vi "Cycling_No_DAQ_Tasks_No_cRio.vi"() -> ()   [LabVIEW 2020]
uses:
  Drivers-IT-M3400/IT-M3400.lvlib
panel:
  in  "Output Safety":T1
  in  "Number of Cycles":i32
  in  "Charge filepath":path
  in  "Discharge filepath":path
  in  "Batteryname":string
  in  "Starting Cycle":i32
  out "PS error out":errorcluster
  out "PS Visa Out":refnum<visa-resource-name>
  in  "Wait time":dbl
  in  "Discharge Current Setpoint":dbl format="%#.6g"
  in  "Charge Current Setpoint":dbl format="%#.6g"
  in  "Battery Type":T2(ring)
  in  "PS type":enum16{"NHR", "ITECH"}(ring)
  in  "PS error in":errorcluster caption="PS error in (no error)"
  in  "PS VISA in":refnum<visa-resource-name>
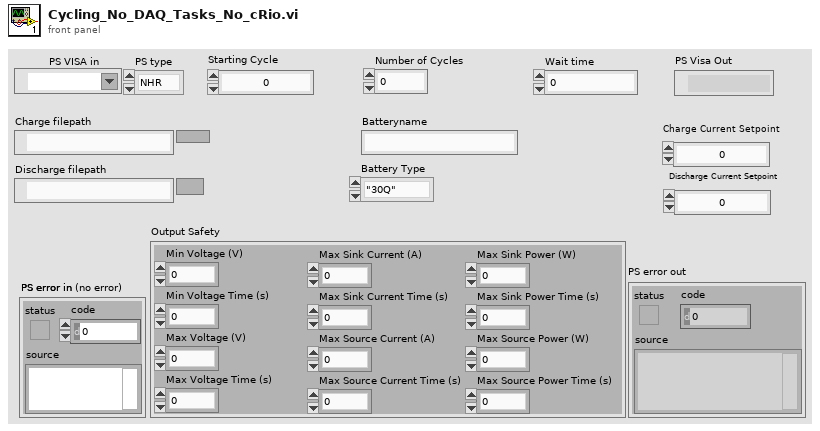
[diagram p1: front panel]
types:
  T1 = cluster{"Min Voltage (V)":dbl, "Min Voltage Time (s)":dbl, "Max Voltage (V)":dbl, "Max Voltage Time (s)":dbl, "Max Sink Current (A)":dbl, "Max Sink Current Time (s)":dbl, "Max Source Current (A)":dbl, "Max Source Current Time (s)":dbl, "Max Sink Power (W)":dbl, "Max Sink Power Time (s)":dbl, "Max Source Power (W)":dbl, "Max Source Power Time (s)":dbl}
  T2 = enum16{"\"30Q\"", "\"40T\"", "\"2P30Q\"", "\"3P30Q\"", "\"Nissan Leaf\""}
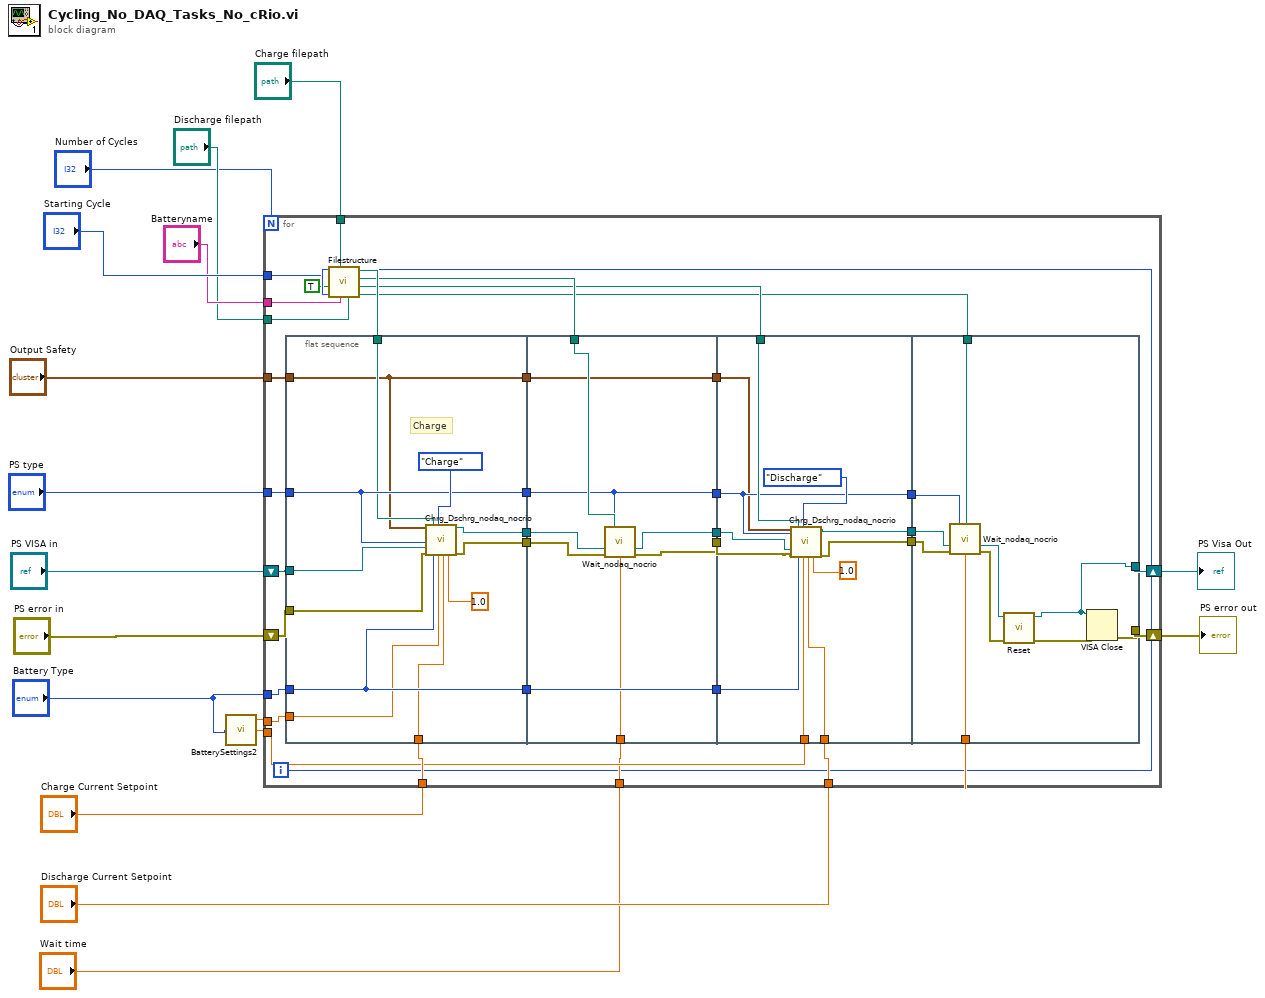
[diagram p0: block diagram]
diagram:
  n1 = call "BatterySettings2.vi"("Battery Type"="Battery Type") -> ("Min Voltage (V)"=w1:dbl, "Max Voltage (V)"=w2:dbl)  [unwired: 2 in, 1 out]
  n2 = for {
    N: "Number of Cycles" -> [_]
    tunnel: "PS type" -> [w42]
    tunnel: w2 -> [w39]
    tunnel: "Battery Type" -> [w38]
    tunnel: "Charge Current Setpoint" -> [w37]
    tunnel: w1 -> [w36]
    tunnel: "Discharge Current Setpoint" -> [w35]
    tunnel: "Wait time" -> [w30]
    shift-right: [w28] -> w10
    shift-left: "PS VISA in" -> [w41]
    shift-right: [w29] -> w11
    shift-left: "PS error in" -> [w40]
    tunnel: "Starting Cycle" -> [w26]
    tunnel: "Batteryname" -> [w24]
    tunnel: "Discharge filepath" -> [w23]
    tunnel: "Charge filepath" -> [w22]
    tunnel: "Output Safety" -> [w20]
    i -> [w27]
    n3 = flat-sequence {
      tunnel: w42 -> [w58]
      tunnel: w41 -> [w61]
      tunnel: w40 -> [w60]
      tunnel: w38 -> [w57]
      tunnel: w39 -> [w56]
      tunnel: w37 -> [w55]
      tunnel: [w62] -> w52
      tunnel: [w63] -> w51
      tunnel: [w58] -> w50
      tunnel: [w57] -> w49
      tunnel: w34 -> [w54]
      tunnel: w20 -> [w53]
      tunnel: [w53] -> w19
      tunnel: w52 -> [w67]
      tunnel: w51 -> [w66]
      tunnel: w50 -> [w68]
      tunnel: [w72] -> w48
      tunnel: [w71] -> w47
      tunnel: [w68] -> w46
      tunnel: w49 -> [w73]
      tunnel: [w73] -> w45
      tunnel: w33 -> [w69]
      tunnel: w30 -> [w70]
      tunnel: w19 -> [w65]
      tunnel: [w65] -> w18
      tunnel: w48 -> [w81]
      tunnel: w47 -> [w80]
      tunnel: w46 -> [w77]
      tunnel: w45 -> [w78]
      tunnel: w36 -> [w79]
      tunnel: w35 -> [w75]
      tunnel: w32 -> [w82]
      tunnel: [w84] -> w44
      tunnel: [w85] -> w43
      tunnel: [w77] -> w21
      tunnel: w18 -> [w74]
      tunnel: w31 -> [w86]
      tunnel: w44 -> [w92]
      tunnel: w43 -> [w91]
      tunnel: w30 -> [w87]
      tunnel: [w95] -> w29
      tunnel: [w94] -> w28
      tunnel: w21 -> [w90]
      frame #0 {
        # "Charge"
        n4 = call "Chrg_Dschrg_nodaq_nocrio.vi"("Output Safety"=w53, "PS type"=w58, "PS VISA in"=w61, "PS error in"=w60, "CyclePath"=w54, "Battery Type"=w57, "Charge/discharge"=enum8{"Charge", "Discharge"}."Charge", "Charge/Discharge Voltage Setpoint"=w56, "Current Setpoint"=w55, "Current Cutoff"=1.0) -> ("PS VISA out"=w62:refnum<visa-resource-name>, "PS error out"=w63:errorcluster)  [unwired: 8 in]
      }
      frame #1 {
        n5 = call "Wait_nodaq_nocrio.vi"("PS type"=w68, "PS VISA in"=w67, "PS error in"=w66, "Wait Filepath"=w69, "Wait time"=w70) -> ("PS Visa Out"=w72:refnum<visa-resource-name>, "PS error out"=w71:errorcluster)  [unwired: 9 in]
      }
      frame #2 {
        n6 = call "Chrg_Dschrg_nodaq_nocrio.vi"("Output Safety"=w74, "PS type"=w77, "PS VISA in"=w81, "PS error in"=w80, "CyclePath"=w82, "Battery Type"=w78, "Charge/discharge"=enum8{"Charge", "Discharge"}."Discharge", "Charge/Discharge Voltage Setpoint"=w79, "Current Setpoint"=w75, "Current Cutoff"=1.0) -> ("PS VISA out"=w84:refnum<visa-resource-name>, "PS error out"=w85:errorcluster)  [unwired: 8 in]
      }
      frame #3 {
        n7 = call "Wait_nodaq_nocrio.vi"("PS type"=w90, "PS VISA in"=w92, "PS error in"=w91, "Wait Filepath"=w86, "Wait time"=w87) -> ("PS Visa Out"=w89:refnum<visa-resource-name>, "PS error out"=w88:errorcluster)  [unwired: 9 in]
        n8 = call "Reset.vi"("error in"=w88, "VISA resource name"=w89) -> ("error out"=w93:errorcluster, "VISA resource name out"=w94:refnum<visa-resource-name>)  [unwired: 8 in]
        n9 = VISA Close(VISA resource name=w94, error in (no error)=w93) -> (error out=w95:errorcluster)
      }
    }
    n10 = call "Filestructure.vi"("Discharge filepath"=w23, "Batteryname"=w24, "Charge filepath"=w22, "For loop i"=w27, "In for loop"=TRUE, "Starting Cycle"=w26) -> ("DischargeWaitPath"=w31:path, "DischargeCyclePath"=w32:path, "ChargeWaitPath"=w33:path, "ChargeCyclePath"=w34:path)  [unwired: 1 in, 1 out]
  }
  "PS error out" <- w11
  "PS Visa Out" <- w10
